vi "TiePie.Gen.init.vi"(8 "error in (no error)":errorcluster, 11 "DevIndex":u32) -> (0 "error out":errorcluster, 3 "GenHandle":T1)   [LabVIEW 2014, in "LVTiePie.lvlib"]
uses:
  LVTiePie.lvlib
  TiePie.Gen.handle.ctl
  bin/libtiepie.dll
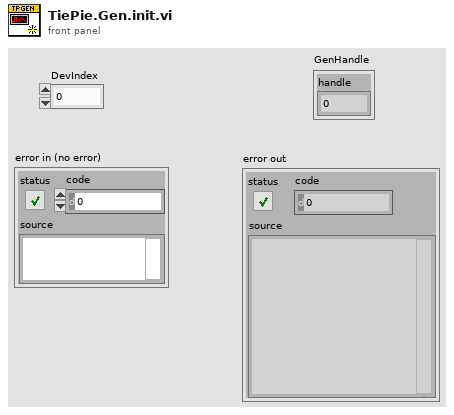
[diagram p1: front panel]
types:
  T1 = typedef "TiePie.Gen.handle.ctl" = cluster{"handle":u32}
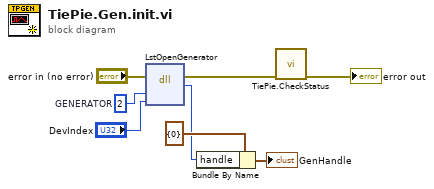
[diagram p0: block diagram]
diagram:
  w8 = u32 2  # GENERATOR
  n1 = dll-call lib="C:/Users/mbirski/Desktop/PAN/LabVEW/Tie Pie/bin/libtiepie.dll" fn="LstOpenGenerator"(error in="error in (no error)", "kind"=w8, "index"="DevIndex") -> (error out=w2:errorcluster, "return type"=w3:u32)  [unwired: 4 in, 1 out]
  n2 = Bundle By Name(cluster=T1 {"handle"=0} ("GenHandle"), "handle"=w3) -> (→"GenHandle":T1)
  n3 = call "TiePie.CheckStatus.vi"("error in (no error)"=w2) -> ("error out"=→"error out":errorcluster)  [unwired: 10 in]
